vi "get c8 peak.vi"() -> (0 "lower limit":dbl, 1 "upper limit":dbl, 2 "laser task out":refnum<k21>, 3 "germanium task out":refnum<k21>)   [LabVIEW 2018]
uses:
  <vilib>/DAQmx/write.llb/DAQmx Write (Analog DBL 1Chan 1Samp).vi
  b68e9a59-4eba-4379-9156-84f4316a9dab.vi
  <vilib>/DAQmx/read.llb/DAQmx Read (Analog DBL 1Chan 1Samp).vi
  <vilib>/Analysis/baseanly.llb/Mean (DBL).vi
  <vilib>/DAQmx/create/channels.llb/DAQmx Create Channel (AO-Voltage-Basic).vi
  <vilib>/DAQmx/miscellaneous.llb/DAQmx Fill In Error Info.vi
  <vilib>/DAQmx/create/channels.llb/DAQmx Create Channel (AI-Voltage-Basic).vi
  <vilib>/ptbypt/NI_PtbyPt.lvlib
  <vilib>/Analysis/NI_AALBase.lvlib
  <vilib>/Analysis/NI_AAL_SigProc.lvlib
panel:
  out "c8 peak (V)":dbl
  in  "sample length":i32=100
  in  "step length (seconds)":dbl=1.0
  out "laser voltage":dbl
  out "diode voltage":dbl
  out "Waveform Chart":cluster{"mean":dbl, "start voltage":dbl}(graph)
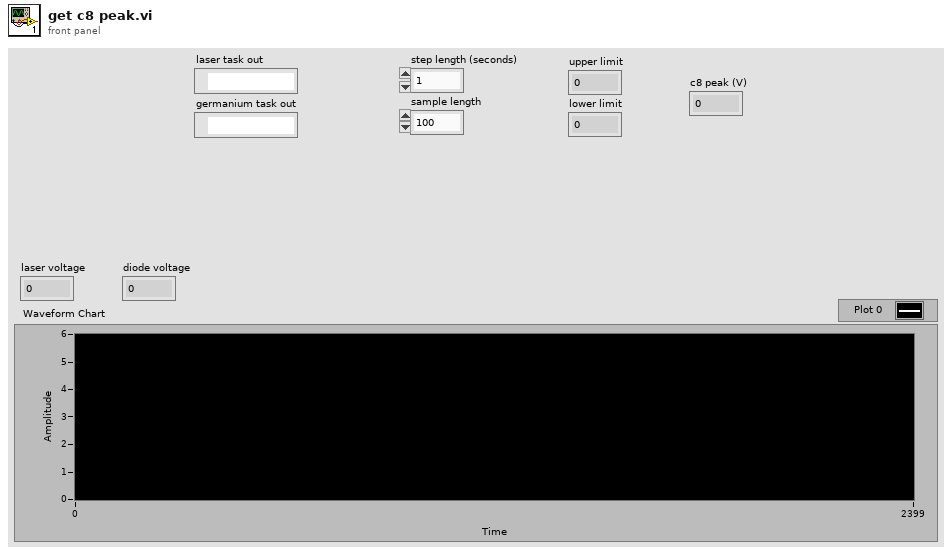
[diagram p1: front panel]
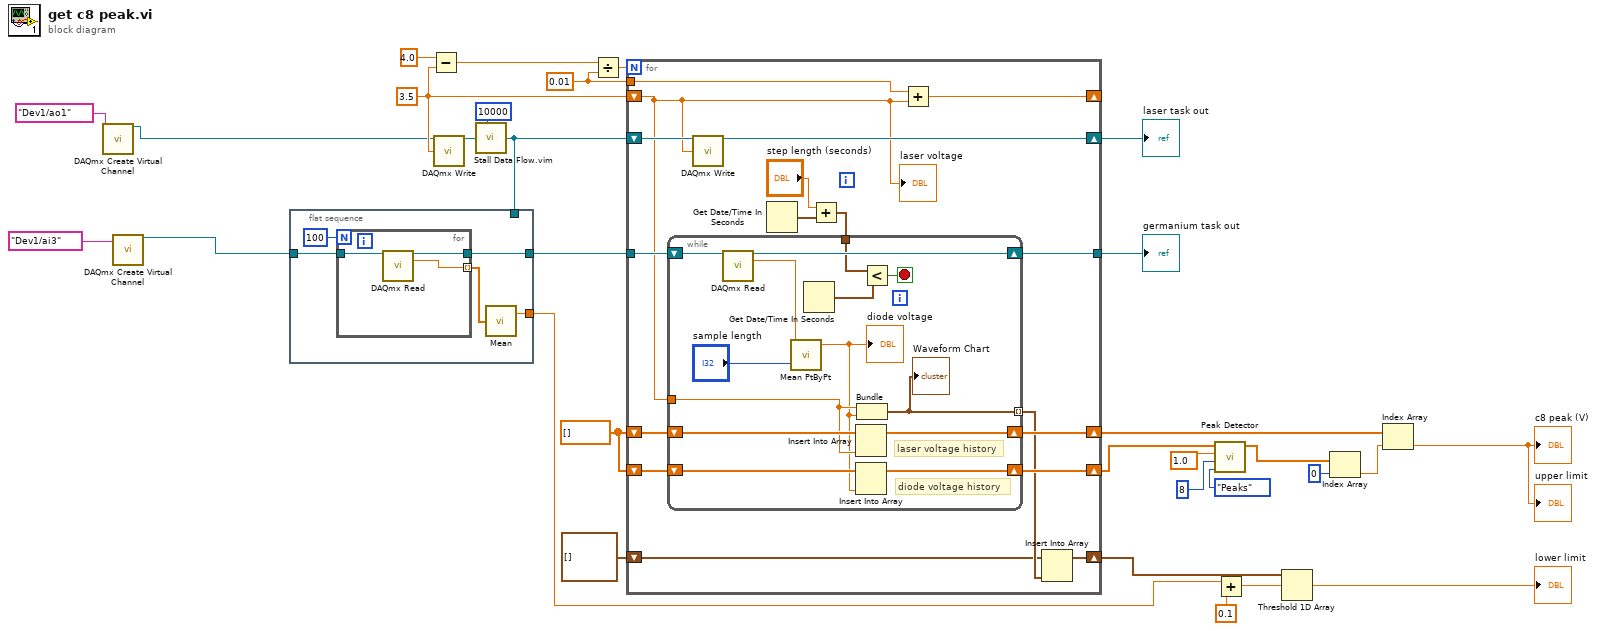
[diagram p0: block diagram]
diagram:
  w25 = 0.01 ("step size")
  w28 = 3.5 ("start voltage")
  w20 = dbl[] []
  n1 = call-poly <vilib>:"DAQmx Create Virtual Channel.vi"("physical channels"=tag "Dev1/ao1") -> ("task out"=w2:refnum<k21>)  [unwired: 13 in, 1 out]
  n2 = call-poly <vilib>:"DAQmx Create Virtual Channel.vi"("physical channels"=tag "Dev1/ai3") -> ("task out"=w1:refnum<k21>)  [unwired: 13 in, 1 out]
  n3 = flat-sequence {
    tunnel: w1 -> [w36]
    tunnel: [w35] -> w22
    tunnel: w21 -> [_]
    tunnel: [w32] -> w7
    frame #0 {
      n4 = for {
        N: 100 -> [_]
        tunnel: [w37] -> w33 mode=indexing
        tunnel: w36 -> [w39]
        tunnel: [w38] -> w35
        n5 = call-poly <vilib>:"DAQmx Read.vi"("task/channels in"=w39) -> ("task out"=w38:refnum<k21>, "data"=w37:dbl)  [unwired: 12 in, 1 out]
      }
      n6 = call-poly <vilib>:"Mean.vi"("X"=w33) -> ("mean"=w32:dbl)  [unwired: 1 out]
    }
  }
  n7 = Subtract(x=4.0 ("end voltage"), y=w28) -> (x-y=w27:dbl)
  n8 = call-poly <vilib>:"DAQmx Write.vi"("task/channels in"=w2, "data"=w28) -> ("task out"=w31:refnum<k21>)  [unwired: 11 in, 2 out]
  n9 = call "Stall Data Flow.vim"("value in"=w31, "milliseconds to wait"=u32 10000) -> ("value out"=w21:refnum<k21>)  [unwired: 1 out]
  n10 = Divide(x=w27, y=w25) -> (x/y=w26:dbl)
  n11 = for {
    N: w26 -> [_]
    shift-right: [w53] -> w24
    shift-left: w21 -> [w56]
    shift-right: [w55] -> _
    shift-left: w28 -> [w50]
    tunnel: w25 -> [w54]
    tunnel: w22 -> [w52]
    tunnel: [w51] -> w23
    shift-right: [w48] -> w10
    shift-left: w20 -> [w49]
    shift-right: [w46] -> w9
    shift-left: w20 -> [w47]
    shift-right: [w44] -> w8
    shift-left: cluster{"start voltage":dbl, "mean":dbl}[] [] -> [w43]
    n12 = call-poly <vilib>:"DAQmx Write.vi"("task/channels in"=w56, "data"=w50) -> ("task out"=w53:refnum<k21>)  [unwired: 11 in, 2 out]
    n13 = Get Date/Time In Seconds() -> (seconds since 1Jan1904=w41:timestamp)
    n14 = Add(x="step length (seconds)", y=w41) -> (x+y=w40:timestamp)
    n15 = while {
      shift-right: [w69] -> w51
      shift-left: w52 -> [w70]
      tunnel: w50 -> [w60]
      shift-right: [w63] -> w48
      shift-left: w49 -> [w64]
      shift-right: [w61] -> w46
      shift-left: w47 -> [w62]
      tunnel: [w58] -> w45 mode=indexing
      tunnel: w40 -> [w57]
      stop <- w66 stop-if-true
      # "laser voltage history"
      # "diode voltage history"
      n16 = call-poly <vilib>:"DAQmx Read.vi"("task/channels in"=w70) -> ("task out"=w69:refnum<k21>, "data"=w67:dbl)  [unwired: 12 in, 1 out]
      n17 = call <vilib>:"Mean PtByPt.vi"("x"=w67, "sample length"="sample length") -> ("mean"=w59:dbl)  [unwired: 2 in, 1 out]
      "diode voltage" <- w59
      n18 = Get Date/Time In Seconds() -> (seconds since 1Jan1904=w65:timestamp)
      n19 = Insert Into Array(array=w64, new element=w60) -> (w63:dbl[])  [unwired: 1 in]
      n20 = Insert Into Array(array=w62, new element=w59) -> (w61:dbl[])  [unwired: 1 in]
      n21 = Bundle("start voltage"=w60, "mean"=w59) -> (w58:cluster{"start voltage":dbl, "mean":dbl})  [unwired: 1 in]
      "Waveform Chart" <- w58
      n22 = Less?(x=w57, y=w65) -> (x < y?=w66:bool)
    }
    n23 = Add(x=w54, y=w50) -> (x+y=w55:dbl)
    n24 = Insert Into Array(array=w43, new element=w45) -> (w44:cluster{"start voltage":dbl, "mean":dbl}[])  [unwired: 1 in]
    "laser voltage" <- w50
  }
  "laser task out" <- w24
  "germanium task out" <- w23
  n25 = call <vilib>:"Peak Detector.vi"("peaks/valleys"=enum32{"Peaks", "Valleys"}."Peaks", "width"=8, "threshold"=1.0, "X"=w9) -> ("Locations"=w16:dbl[])  [unwired: 3 in, 4 out]
  n26 = Add(x=w7, y=0.1) -> (x+y=w12:dbl)
  n27 = Threshold 1D Array(2:w12, 3:w8) -> (0:→"lower limit":dbl)  [unwired: 1 in]
  n28 = Index Array(array=w16, index=0) -> (element=w14:dbl)
  n29 = Index Array(array=w10, index=w14) -> (element=→"c8 peak (V)" →"upper limit":dbl)
